vi "FET_vs_DRAIN.vi"() -> ()   [LabVIEW 2014]
doc: "FET1 = I_DS vs V_DS\nMisura la caratteristica di un FET canale N\nfissando V sul DRAIN e variando V _GATE\nFM & ADL 2015/11"
uses:
  <vilib>/DAQmx/write.llb/DAQmx Write (Analog DBL 1Chan 1Samp).vi
  <vilib>/DAQmx/create/channels.llb/DAQmx Create Channel (AO-Voltage-Basic).vi
  <vilib>/DAQmx/configure/timing.llb/DAQmx Timing (Sample Clock).vi
  <vilib>/DAQmx/miscellaneous.llb/DAQmx Fill In Error Info.vi
  <vilib>/Utility/file.llb/Write To Spreadsheet File (DBL).vi
panel:
  in  "R_SOURCE (kOhm)":dbl=0.1 format="%_4g"
  in  "V_GATE":dbl=4.0 min=-10.0 max=10.0 step=0.025 format="%.3f"
  in  "Fondo Scala AI1":dbl(ring)=5.0 items=["10"=10.0, "5"=5.0, "0.5"=0.5, "0.05"=0.05]
  in  "SALVA I DATI":bool=TRUE caption="ON\nOFF"
  out "V_DRAIN":dbl=1.0 format="%_3g"
  out "No Misura":i32=25
  in  "Fondo Scala AI0":dbl(ring)=10.0 items=["10"=10.0, "5"=5.0, "0.5"=0.5, "0.05"=0.05]
  out "Corrente DRAIN-SOURCE in funzione della V_DS":cluster{dbl[], dbl[]}(graph)={[0.0001492957157763555, 0.005316779605869654, 0.010282789302859877, 0.015212154519744406, 0.020253928641941782, 0.025218550093194098, 0.030214316848511696, 0.035253225798399845, 0.04064751611193518, 0.04579588182765809, 0.05091598666495806, 0.05624595407868921, 0.06144059627479942, 0.06679958055171675, 0.07239242133010548, 0.07775224012072779, 0.08325257315332713, 0.08877255157285258, 0.09450280540089562, 0.10022008450642927, 0.10645289338765562, 0.11244413683857102, 0.1186399870272482, 0.1250692028788145, 0.13167287017949103], [-0.0014929571577635549, 0.3634988706079701, 0.7305054403047345, 1.097878454802556, 1.4641273802472488, 1.8311478324013921, 2.197856831514883, 2.564134408682668, 2.926858172213981, 3.2920411817234188, 3.6575068000170856, 4.020873792546441, 4.385594037252005, 4.748670861149498, 5.109409120032278, 5.472477598792722, 5.834140935133394, 6.195607817604807, 6.554971945991044, 6.9144658216023736, 7.268804399456776, 7.62555863161429, 7.980266796394184, 8.332641304545186, 8.683271298205089]}
  out "V_SOURCE":dbl=0.868327129820509 format="%_3f"
  in  "# misure":i16=25
  in  "Vmax":dbl=1.0 max=100000.0
  in  "Vmin":dbl
  # "Valore consigliato  R_SOURCE = 100 Ohm"
  # "1) Selezionare il valore minimo e massimo della tensione applicata al DRAIN  ed il numero di valori (equispaziati  tra gli estremi). \nSelezionare la tensione fissa applicata al GATE.\nSelezionare il valore della resistenza in serie al SOURCE."
  # "2) Collegare il CB22 e CB68 al GATE,   \n    CB21 al DRAIN,  \n    CB33 alla resistenza in serie al SOURCE.\nLa terra del circuito DEVE essere in comune alla terra della scheda (CB29)."
  # "Durante la misura gli indicatori mostrano i valori di I_DRAIN,   V_DRAIN , V_SOURCE ed il numero progressivo della misura.\n\nSul grafico viene mostrata la corrente che scorre da DRAIN a SOURCE  in funzione della tensione GATE-SOURCE."
  # "NO\nSI"
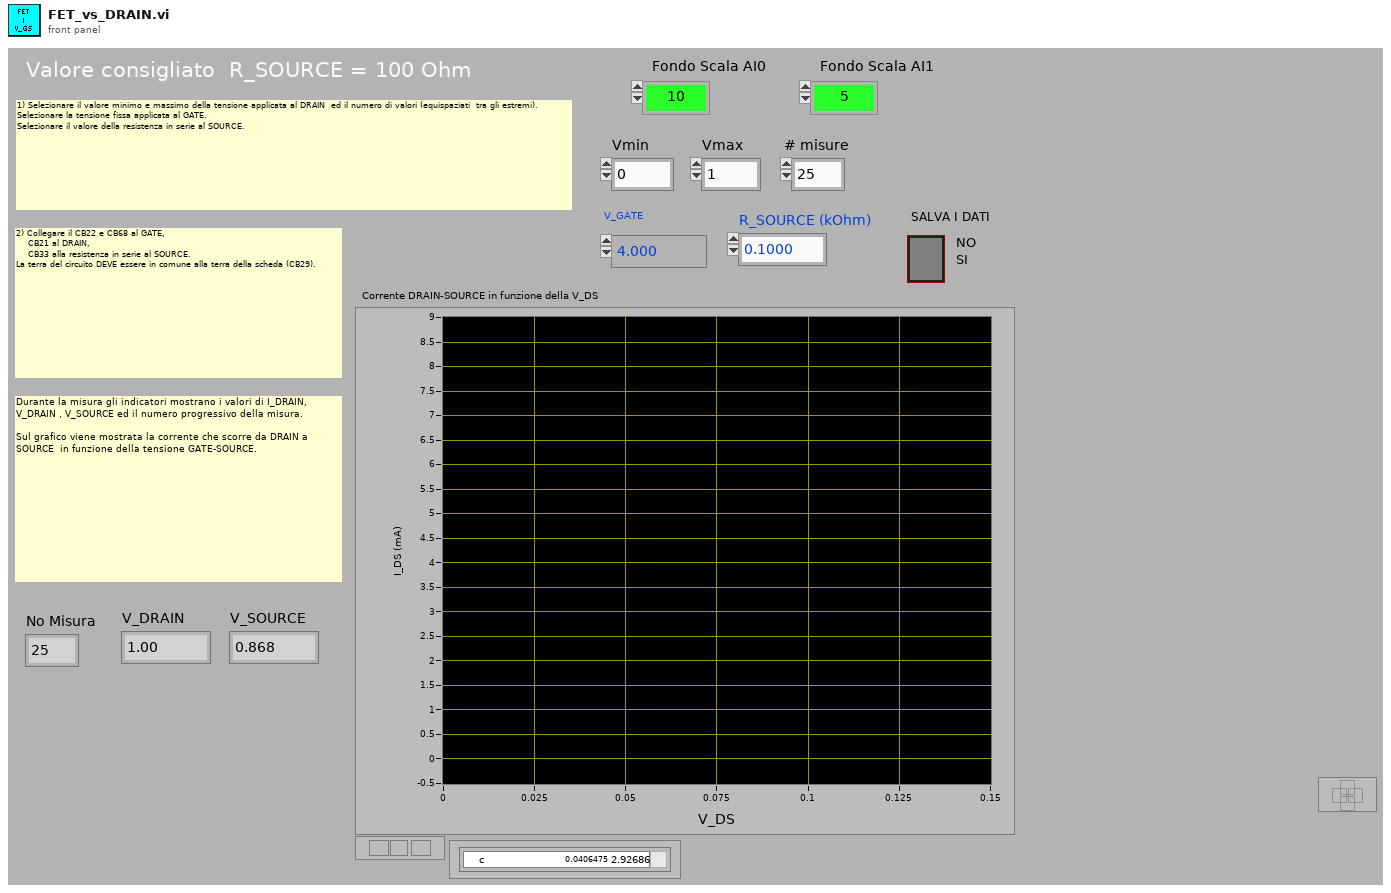
[diagram p1: front panel]
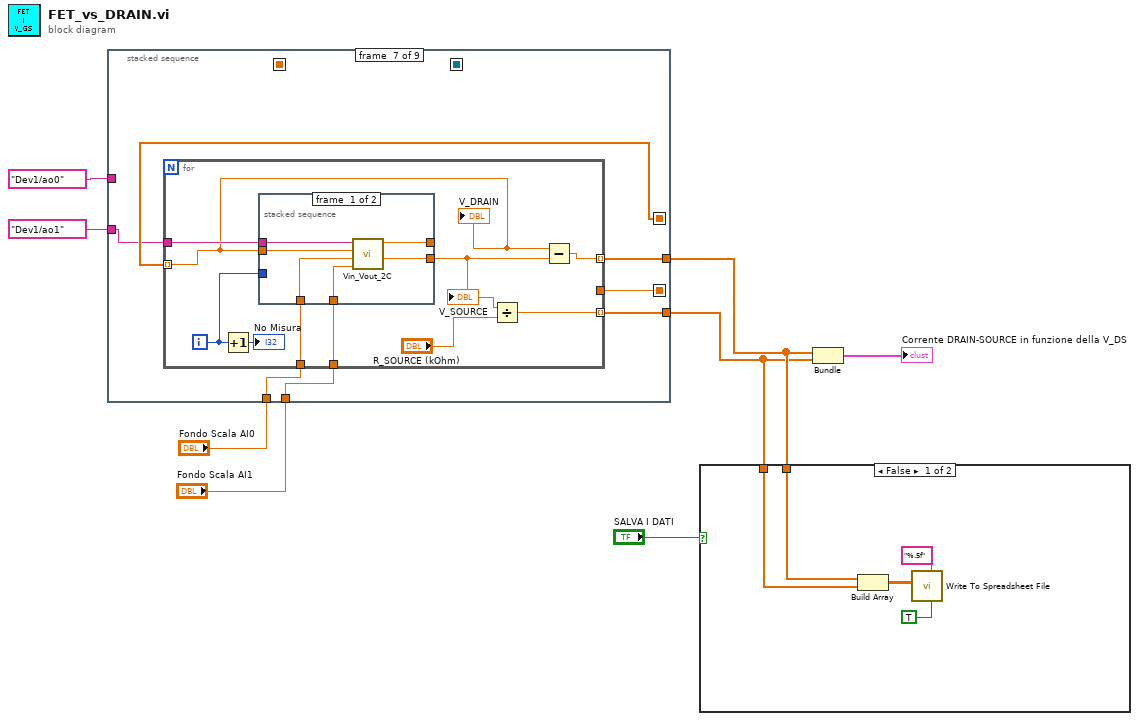
[diagram p0: block diagram]
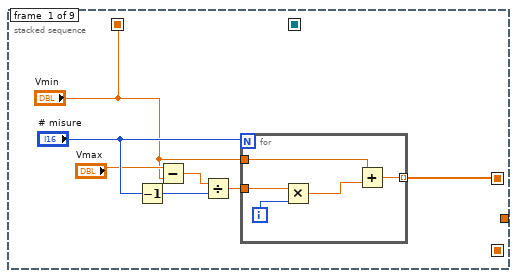
[diagram p3: hidden frame]
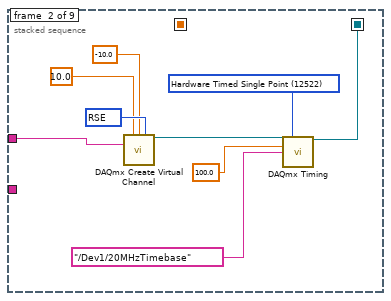
[diagram p4: hidden frame]
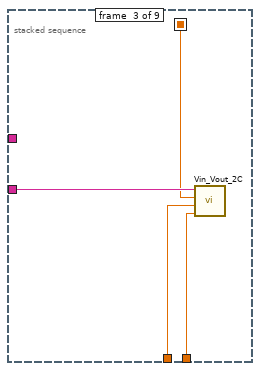
[diagram p5: hidden frame]
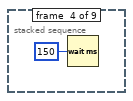
[diagram p6: hidden frame]
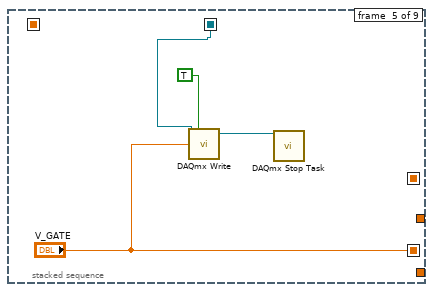
[diagram p7: hidden frame]
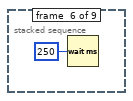
[diagram p8: hidden frame]
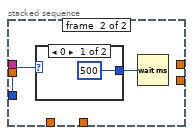
[diagram p9: hidden frame]
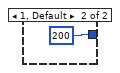
[diagram p10: hidden frame]
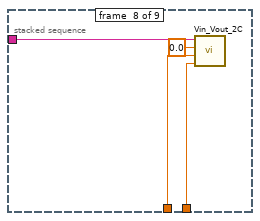
[diagram p11: hidden frame]
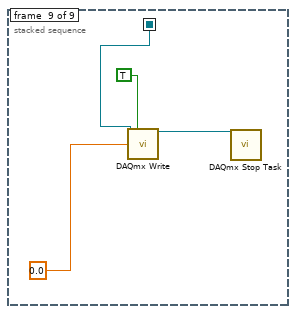
[diagram p12: hidden frame]
diagram:
  n1 = stacked-sequence {
    seq-local: [w12 _ _ _ _ _ _ _ _] -> [_ _ _ _ _ _ w45 _ _]
    seq-local: [_ w22 _ _ _ _ _ _ _] -> [_ _ _ _ w37 _ _ _ w73]
    seq-local: [_ _ _ _ "V_GATE" _ _ _ _] -> [_ _ _ _ _ _ w40 _ _]
    seq-local: ["Vmin" _ _ _ _ _ _ _ _] -> [_ _ w30 _ _ _ _ _ _]
    tunnel: "Fondo Scala AI1" -> [_ _ w31 _ _ _ w46 w68 _]
    tunnel: "Fondo Scala AI0" -> [_ _ w32 _ _ _ w44 w69 _]
    tunnel: tag "Dev1/ao0" ("physical channels") -> [_ w21 _ _ _ _ _ _ _]
    tunnel: tag "Dev1/ao1" ("physical channels") -> [_ _ w33 _ _ _ w43 w70 _]
    tunnel: [_ _ _ _ _ _ w42 _ _] -> w1
    tunnel: [_ _ _ _ _ _ w41 _ _] -> w2
    frame #0 {
      n2 = Decrement(x="# misure") -> (x-1=w14:i16)
      n3 = Subtract(x="Vmax", y="Vmin") -> (x-y=w15:dbl)
      n4 = Divide(x=w15, y=w14) -> (x/y=w13:dbl)
      n5 = for {
        N: "# misure" -> [_]
        tunnel: "Vmin" -> [w20]
        tunnel: [w19] -> w12 mode=indexing
        tunnel: w13 -> [w18]
        i -> [w17]
        n6 = Multiply(x=w18, y=w17) -> (x*y=w16:dbl)
        n7 = Add(x=w20, y=w16) -> (x+y=w19:dbl)
      }
    }
    frame #1 {
      w26 = 12522 items=["Finite Samples"=10178, "Continuous Samples"=10123, "Hardware Timed Single Point"=12522] ("sample mode")
      w29 = 10083 items=["Default"=-1, "RSE"=10083, "Differential"=10106, "Pseudodifferential"=12529] ("output terminal configuration")
      n8 = call-poly <vilib>:"DAQmx Create Virtual Channel.vi"("maximum value"=10.0, "minimum value"=-10.0, "output terminal configuration"=w29, "physical channels"=w21) -> ("task out"=w24:refnum<k21>)  [unwired: 5 in, 6 out]
      n9 = call-poly <vilib>:"DAQmx Timing.vi"("task/channels in"=w24, "sample mode"=w26, "rate"=100.0, "source"=tag "/Dev1/20MHzTimebase") -> ("task out"=w22:refnum<k21>)  [unwired: 3 in, 8 out]
    }
    frame #2 {
      n10 = call "Vin_Vout_2C.vi"("Fondo Scala AI1 (33)"=w31, "Fondo Scala AI0 (68)"=w32, "V in volt"=w30, "Canale uscita"=w33) -> ()  [unwired: 4 out]
    }
    frame #3 {
      n11 = Wait (ms)(milliseconds to wait=u32 150) -> ()  [unwired: 1 out]
    }
    frame #4 {
      n12 = call-poly <vilib>:"DAQmx Write.vi"("task/channels in"=w37, "auto start"=TRUE, "data"="V_GATE") -> ("task out"=w36:refnum<k21>)  [unwired: 1 in, 11 out]
      n13 = call <vilib>:"DAQmx Stop Task.vi"("task/channels in"=w36) -> ()  [unwired: 1 in, 14 out]
    }
    frame #5 {
      n14 = Wait (ms)(milliseconds to wait=u32 250) -> ()  [unwired: 1 out]
    }
    frame #6 {
      n15 = for {
        tunnel: w45 -> [w47] mode=indexing
        tunnel: w46 -> [w56]
        tunnel: w44 -> [w54]
        tunnel: w43 -> [w52]
        tunnel: [w48] -> w42 mode=indexing
        tunnel: [w51] -> w41 mode=indexing
        tunnel: w40 -> [_]
        i -> [w53]
        n16 = Increment(x=w53) -> (x+1=→"No Misura":i32)
        n17 = stacked-sequence {
          tunnel: w47 -> [w60 _]
          tunnel: w56 -> [w61 _]
          tunnel: w54 -> [w62 _]
          tunnel: w53 -> [_ w63]
          tunnel: w52 -> [w59 _]
          tunnel: [w58 _] -> _
          tunnel: [w57 _] -> w50
          frame #0 {
            n18 = call "Vin_Vout_2C.vi"("Fondo Scala AI1 (33)"=w61, "Fondo Scala AI0 (68)"=w62, "V in volt"=w60, "Canale uscita"=w59) -> ("V1 medio"=w57:dbl, "V0 medio"=w58:dbl)  [unwired: 2 out]
          }
          frame #1 {
            n19 = case shown="0" w63 {
              tunnel: [500 u32 200 ("milliseconds to wait")] -> w64
              frame 0 {
              }
              frame 1, Default {
              }
            }
            n20 = Wait (ms)(milliseconds to wait=w64) -> ()  [unwired: 1 out]
          }
        }
        "V_SOURCE" <- w50
        n21 = Divide(x=w50, y="R_SOURCE (kOhm)") -> (x/y=w48:dbl)
        n22 = Subtract(x=w47, y=w50) -> (x-y=w51:dbl)
        "V_DRAIN" <- w47
      }
    }
    frame #7 {
      n23 = call "Vin_Vout_2C.vi"("Fondo Scala AI1 (33)"=w68, "Fondo Scala AI0 (68)"=w69, "V in volt"=0.0, "Canale uscita"=w70) -> ()  [unwired: 4 out]
    }
    frame #8 {
      n24 = call-poly <vilib>:"DAQmx Write.vi"("task/channels in"=w73, "auto start"=TRUE, "data"=0.0) -> ("task out"=w71:refnum<k21>)  [unwired: 1 in, 11 out]
      n25 = call <vilib>:"DAQmx Stop Task.vi"("task/channels in"=w71) -> ()  [unwired: 1 in, 14 out]
    }
  }
  n26 = case shown="False" "SALVA I DATI" {
    tunnel: w2 -> [w79 _]
    tunnel: w1 -> [w78 _]
    frame False {
      n27 = Build Array(w79, w78) -> (w75:dbl[][])
      n28 = call-poly <vilib>:"Write To Spreadsheet File.vi"("transpose? (no:F)"=TRUE, "format (%.3f)"="%.5f", "2D data"=w75) -> ()  [unwired: 3 in, 3 out]
    }
    frame True {
    }
  }
  n29 = Bundle(w2, w1) -> (→"Corrente DRAIN-SOURCE in funzione della V_DS":cluster{dbl[], dbl[]})  [unwired: 1 out]
